vi "libssh2_sftp_fstatvfs.vi"(8 "error in (no error)":errorcluster, 11 "sftp handle":T2) -> (0 "error out":errorcluster, 2 "statvfs":T1)   [LabVIEW 2013, in "libssh2.lvlib"]
doc: "Get the file system information of a file handle."
uses:
  libssh2.lvlib
  SFTP Handle Refnum.ctl
  libssh2_sftp_statvfs.ctl
  Not An SFTP Handle Refnum.vi
  <vilib>/Utility/error.llb/Error Cluster From Error Code.vi
  Global Settings.vi
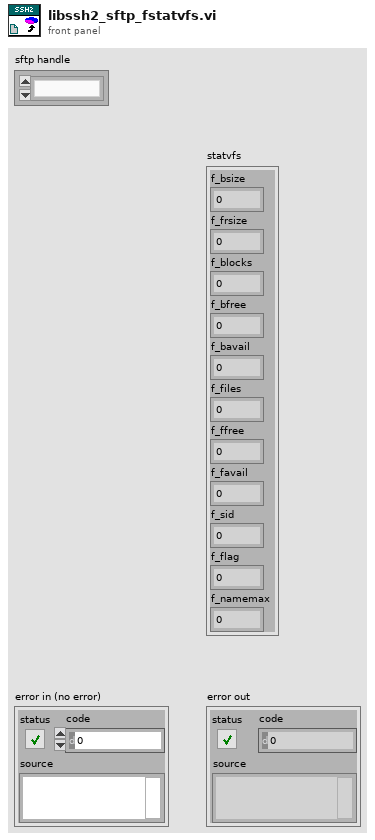
[diagram p1: front panel]
types:
  T1 = typedef "libssh2.lvlib/libssh2_sftp_statvfs.ctl" = cluster{"f_bsize":u64, "f_frsize":u64, "f_blocks":u64, "f_bfree":u64, "f_bavail":u64, "f_files":u64, "f_ffree":u64, "f_favail":u64, "f_sid":u64, "f_flag":u64, "f_namemax":u64}
  T2 = typedef "libssh2.lvlib/SFTP Handle Refnum.ctl" = refnum<k1>
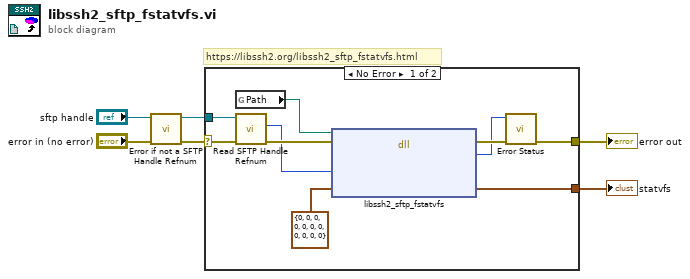
[diagram p0: block diagram]
diagram:
  # "https://libssh2.org/libssh2_sftp_fstatvfs.html"
  n1 = call "Error if not a SFTP Handle Refnum.vi"("error in (no error)"="error in (no error)", "sftp handle"="sftp handle") -> ("error out"=w5:errorcluster, "sftp handle out"=w4:T2)  [unwired: 8 in]
  n2 = case shown="No Error" w5 {
    selector: w5 -> [w15 w17]
    tunnel: w4 -> [w14 _]
    tunnel: [w10 w17] -> w3
    tunnel: [w7 _] -> w1
    frame No Error {
      n3 = global read "Global Settings.vi" "Path"() -> (w16:path)
      n4 = call "Read SFTP Handle Refnum.vi"("error in (no error)"=w15, "sftp handle"=w14) -> ("error out"=w13:errorcluster, "LIBSSH2_SFTP_HANDLE*"=w12:u64)  [unwired: 8 in]
      n5 = dll-call lib="?" fn="libssh2_sftp_fstatvfs"(path in=w16, error in=w13, "handle"=w12, "st"=T1 {"f_bsize"=0, "f_frsize"=0, "f_blocks"=0, "f_bfree"=0, "f_bavail"=0, "f_files"=0, "f_ffree"=0, "f_favail"=0, "f_sid"=0, "f_flag"=0, "f_namemax"=0} ("statvfs")) -> (error out=w11:errorcluster, "return value"=w9:i32, "st"=w7:T1)  [unwired: 2 in, 1 out]
      n6 = call "Error Status.vi"("error in (no error)"=w11, "return value"=w9) -> ("error out"=w10:errorcluster)  [unwired: 8 in, 1 out]
    }
    frame Error {
    }
  }
  "error out" <- w3
  "statvfs" <- w1
